vi "Generate Unique Header.vi"(8 "error in (no error)":errorcluster, 11 "PPT Data in":refnum<class "PPT Data.lvclass">) -> (0 "error out":errorcluster, 2 "Header":string[](array[string]), 3 "PPT Data out":refnum<class "PPT Data.lvclass">)   [LabVIEW 2014, in "PPT Library.lvlib" / "PPT Data.lvclass"]
uses:
  PPT Data.lvclass
  reusable/Data/Data.lvclass/Data.ctl
  reusable/Data/Read Data ID.vi
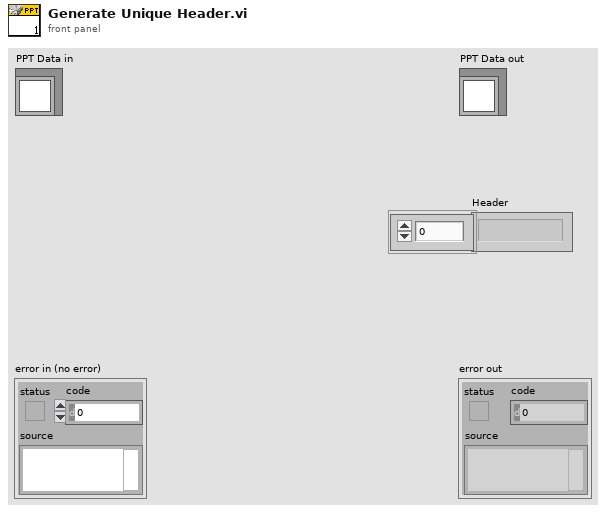
[diagram p1: front panel]
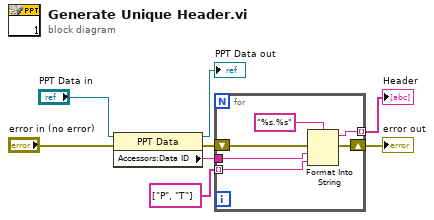
[diagram p0: block diagram]
diagram:
  n1 = property class="PPT Data"(reference="PPT Data in", error in="error in (no error)") -> (reference out=→"PPT Data out":refnum<class "PPT Data.lvclass">, error out=w2:errorcluster, "Accessors:Data ID"=w4:string)
  n2 = for {
    tunnel: string[] ["P", "T"] -> [w13] mode=indexing
    tunnel: w4 -> [w12]
    tunnel: [w11] -> w3 mode=indexing
    shift-right: [w9] -> w1
    shift-left: w2 -> [w10]
    n3 = Format Into String(format string="%s.%s", error in=w10, w12, w13) -> (resulting string=w11:string, error out=w9:errorcluster)  [unwired: 1 in]
  }
  "error out" <- w1
  "Header" <- w3
